vi "Test VI.vi"   [LabVIEW 2016, in "SLL Class DVR API Generator.lvlib"]
uses:
  SLL Class DVR API Generator.lvlib
  Example/My Sample Class.lvclass
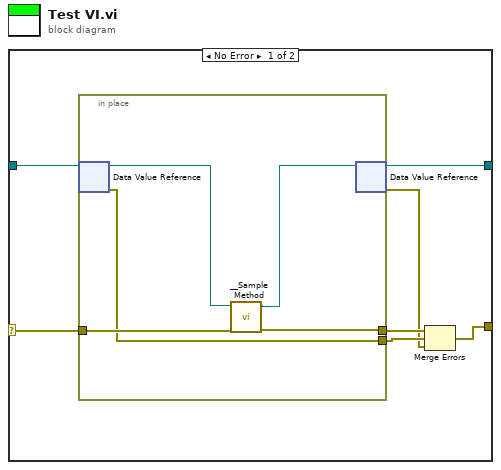
[diagram p0: block diagram]
diagram:
  n1 = case "Error Case Structure" shown="No Error" {
    selector: _ -> [w7 w14]
    tunnel: [w5 w14] -> _
    tunnel: _ -> [w4 w13]
    tunnel: [w3 w13] -> _
    frame No Error {
      n2 = in-place "DVR In Place Element Structure" {
        in-place-border: w7 -> [w9]
        in-place-border: [w12] -> w6
        in-place-border: [w8] -> w2
        n3 = in-place-dvr #1(w4) -> (w11:refnum<class "My Sample Class.lvclass">, w8:errorcluster)
        n4 = call "__Sample Method.vi"("error in (no error)"=w9, "My Sample Class in"=w11) -> ("error out"=w12:errorcluster, "My Sample Class out"=w10:refnum<class "My Sample Class.lvclass">)  [unwired: 8 in]
        n5 = in-place-dvr #1(w10) -> (w3:refnum<data-value>, w1:errorcluster)
      }
      n6 = Merge Errors(w6, w2, w1) -> (w5:errorcluster)
    }
    frame Error {
    }
  }
